vi "Memory.Pointer.Write (safe).vi"(8 "error in (no error)":errorcluster, 9 "offset (0)":u64 format="%d bytes", 10 "data":string, 11 "Pointer in":refnum<class "Memory.Pointer.lvclass">) -> (0 "error out":errorcluster, 1 "offset dup":u64 format="%d bytes", 2 "data dup":string, 3 "Pointer out":refnum<class "Memory.Pointer.lvclass">)   [LabVIEW 2016, in "LabVIEW Memory Manager.lvlib" / "Memory.Pointer.lvclass"]
uses:
  Memory.Pointer.lvclass
  Memory.Pointer.lvclass/Memory.Pointer.ctl
  Accessors/Memory.Pointer.Get Address.vi
  LabVIEW Memory Manager.lvlib
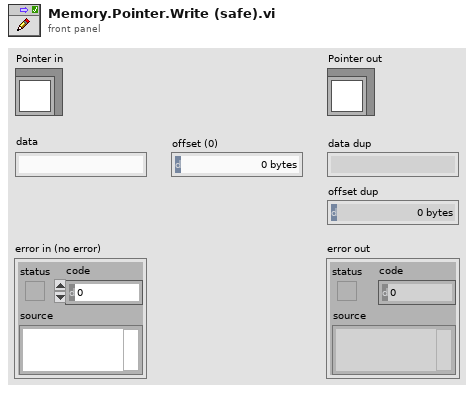
[diagram p1: front panel]
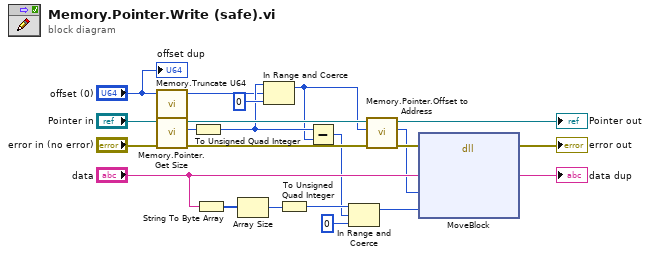
[diagram p0: block diagram]
diagram:
  n1 = call "Memory.Truncate U64.vi"("U64"="offset (0)") -> ("truncated U64"=w2:u64)  [unwired: 10 in]
  n2 = call "Memory.Pointer.Get Size.vi"("error in (no error)"="error in (no error)", "Pointer in"="Pointer in") -> ("error out"=w11:errorcluster, "size"=w15:i64, "Pointer out"=w12:refnum<class "Memory.Pointer.lvclass">)  [unwired: 7 in]
  n3 = To Unsigned Quad Integer(1:w15) -> (0:w10:u64)
  n4 = String To Byte Array(string="data") -> (unsigned byte array=w22:u8[])
  n5 = Array Size(array=w22) -> (size(s)=w9:i32)
  n6 = In Range and Coerce(upper limit=w10, x=w2, lower limit=u64 0) -> (coerced(x)=w4:u64)  [unwired: 1 out]
  n7 = To Unsigned Quad Integer(1:w9) -> (0:w7:u64)
  n8 = Subtract(x=w10, y=w4) -> (x-y=w6:u64)
  n9 = In Range and Coerce(upper limit=w7, x=w6, lower limit=u64 0) -> (coerced(x)=w5:u64)  [unwired: 1 out]
  n10 = call "Memory.Pointer.Offset to Address.vi"("error in (no error)"=w11, "offset"=w4, "Pointer in"=w12) -> ("error out"=w18:errorcluster, "address"=w17:u64, "Pointer out"=→"Pointer out":refnum<class "Memory.Pointer.lvclass">)  [unwired: 5 in, 1 out]
  n11 = dll-call lib="LabVIEW" fn="MoveBlock"(error in=w18, "src pointer"="data", "dst pointer"=w17, "size"=w5) -> (error out=→"error out":errorcluster, "src pointer"=→"data dup":string)  [unwired: 5 in, 1 out]
  "offset dup" <- "offset (0)"
